vi "Stream to Text File - 1 channel 1 sample.vi"() -> ()   [LabVIEW 2020]
uses:
  <vilib>/DAQmx/miscellaneous.llb/DAQmx Fill In Error Info.vi
  <vilib>/DAQmx/read.llb/DAQmx Read (Analog DBL 1Chan 1Samp).vi
  <vilib>/DAQmx/configure/timing.llb/DAQmx Timing (Sample Clock).vi
  <vilib>/DAQmx/create/channels.llb/DAQmx Create Channel (AI-Temperature-Thermocouple).vi
panel:
  out "Waveform Chart":dbl(graph)=61.68840446814595
  in  "minimum value":dbl
  in  "maximum value":dbl=100.0
  in  "Thermocouple Channel":tag="PCI-6221/ai1"
  in  "stop":bool
  # "Measurement Range"
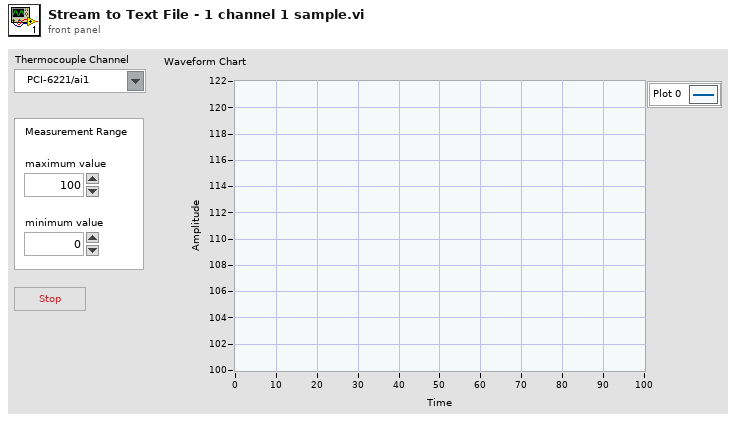
[diagram p1: front panel]
types:
  T1 = enum16{"open", "replace", "create", "open or create", "replace or create", "replace or create with confirmation"}
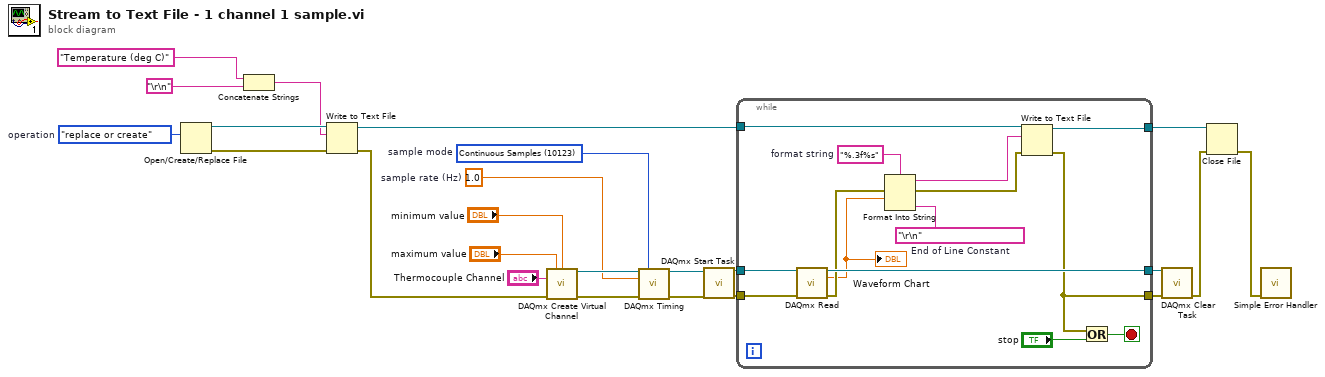
[diagram p0: block diagram]
diagram:
  w10 = T1."replace or create"  # operation
  w19 = 1.0  # sample rate (Hz)
  w20 = 10123 items=["Finite Samples"=10178, "Continuous Samples"=10123, "Hardware Timed Single Point"=12522]  # sample mode
  n1 = Open/Create/Replace File(operation (0:open)=w10) -> (refnum out=w12:refnum<file>, error out=w11:errorcluster)  [unwired: 5 in, 1 out]
  n2 = Concatenate Strings "Concatenate Strings"("Temperature (deg C)", "\r\n") -> (w7:string)
  n3 = Write to Text File(file (use dialog)=w12, text=w7, error in=w11) -> (refnum out=w13:refnum<file>, error out=w14:errorcluster)  [unwired: 1 in, 1 out]
  n4 = call-poly <vilib>:"DAQmx Create Virtual Channel.vi"("maximum value"="maximum value", "minimum value"="minimum value", "physical channels"="Thermocouple Channel", "error in"=w14) -> ("task out"=w24:refnum<k21>, "error out"=w23:errorcluster)  [unwired: 10 in]
  n5 = call-poly <vilib>:"DAQmx Timing.vi"("task/channels in"=w24, "sample mode"=w20, "rate"=w19, "error in"=w23) -> ("task out"=w18:refnum<k21>, "error out"=w17:errorcluster)  [unwired: 10 in]
  n6 = call <vilib>:"DAQmx Start Task.vi"("task/channels in"=w18, "error in"=w17) -> ("task out"=w22:refnum<k21>, "error out"=w21:errorcluster)  [unwired: 12 in]
  n7 = while {
    tunnel: w22 -> [w38]
    tunnel: w21 -> [w37]
    tunnel: [w36] -> w16
    tunnel: [w27] -> w15
    tunnel: w13 -> [w34]
    tunnel: [w33] -> w6
    stop <- w35 stop-if-true
    w30 = "\r\n"  # End of Line Constant
    w32 = "%.3f%s"  # format string
    n8 = call-poly <vilib>:"DAQmx Read.vi"("task/channels in"=w38, "error in"=w37) -> ("task out"=w36:refnum<k21>, "data"=w25:dbl, "error out"=w31:errorcluster)  [unwired: 11 in]
    "Waveform Chart" <- w25
    n9 = Format Into String "Format Into String"(format string=w32, error in=w31, w25, w30) -> (resulting string=w29:string, error out=w28:errorcluster)  [unwired: 1 in]
    n10 = Write to Text File(file (use dialog)=w34, text=w29, error in=w28) -> (refnum out=w33:refnum<file>, error out=w27:errorcluster)  [unwired: 1 in, 1 out]
    n11 = Or(x=w27, y="stop") -> (x .or. y?=w35:bool)
  }
  n12 = call <vilib>:"DAQmx Clear Task.vi"("task in"=w16, "error in"=w15) -> ("error out"=w5:errorcluster)  [unwired: 13 in]
  n13 = Close File(refnum=w6, error in=w5) -> (error out=w4:errorcluster)  [unwired: 1 out]
  n14 = call <vilib>:"Simple Error Handler.vi"("error in (no error)"=w4) -> ()  [unwired: 4 in, 5 out]
